vi "EditOptions.vi"(8 "error in":errorcluster, 11 "Fgen Instrument":refnum<class "Fgen Instrument.lvclass">) -> (0 "error out":errorcluster, 1 "edit options":T1, 2 "subnodes class":T2, 3 "Fgen Instrument out":refnum<class "Fgen Instrument.lvclass">)   [LabVIEW 2025, in "Fgen.lvlib" / "Fgen Instrument.lvclass"]
doc: "This VI Contains the options for the Menu that will be displayed when doing right click on an item\nThe subnodes class configures which nodes can be added to this nodes\nAnd the edit options determine which options are available for the node.\n\nThis configuration is stored in this VI in case some dynamic configuration is required for the menu options or subnodes.\n\nAll VIs must overide this methodCopyright 2017 National Instruments Corporation\n\nLicensed under the Apache License, Version 2.0 (the \"License\"); you may not use this file except in compliance with the License. You may obtain a copy of the License at http://www.apache.org/licenses/LICENSE-2.0\nUnless required by applicable law or agreed to in writing, software distributed under the License is distributed on an \"AS IS\" BASIS, WITHOUT WARRANTIES OR CONDITIONS OF ANY KIND, either express or implied. See the License for the specific language governing permissions and limitations under the License."
uses:
  Fgen Instrument.lvclass
  Users/Public/Documents/Sandia National Labs/TSS Plugin/CEF.lvlibp/Node/SubNodeCluster.ctl
  Users/Public/Documents/Sandia National Labs/TSS Plugin/CEF.lvlibp/Node/NodeMenuOptions.ctl
  Users/Public/Documents/Sandia National Labs/TSS Plugin/CEF.lvlibp/Node/CEF_Node.lvclass
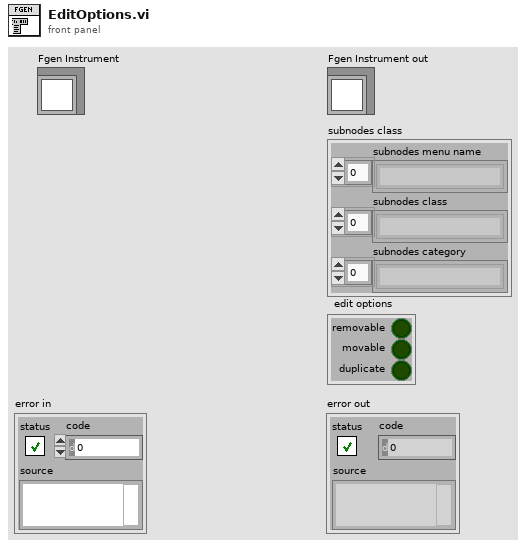
[diagram p1: front panel]
types:
  T1 = typedef "CEF.lvlibp/CEF_Node.lvclass/NodeMenuOptions.ctl" = cluster{"removable":bool, "movable":bool, "duplicate":bool}
  T2 = typedef "CEF.lvlibp/CEF_Node.lvclass/SubNodeCluster.ctl" = cluster{"subnodes menu name":string[], "subnodes class":string[], "subnodes category":string[]}
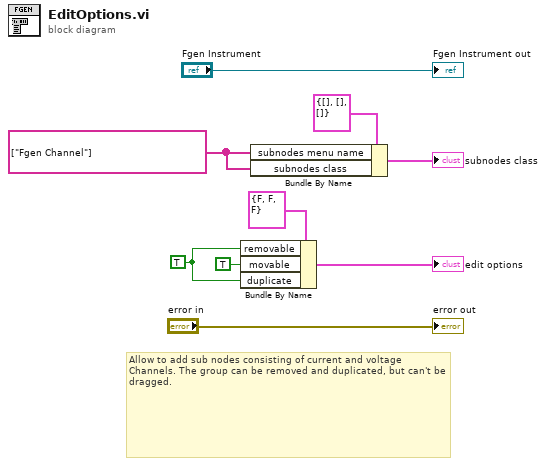
[diagram p0: block diagram]
diagram:
  w7 = TRUE ("movable")
  w2 = string[] ["Fgen Channel"] ("subnodes class")
  # "Allow to add sub nodes consisting of current and voltage Channels. The group can be removed and duplicated, but can't be dragged."
  n1 = Bundle By Name(cluster=T1 {"removable"=FALSE, "movable"=FALSE, "duplicate"=FALSE} ("edit options 2"), "removable"=w7, "movable"=TRUE, "duplicate"=w7) -> (→"edit options":T1)
  n2 = Bundle By Name(cluster=T2 {"subnodes menu name"=[], "subnodes class"=[], "subnodes category"=[]} ("subnodes class"), "subnodes menu name"=w2, "subnodes class"=w2) -> (→"subnodes class":T2)
  "error out" <- "error in"
  "Fgen Instrument out" <- "Fgen Instrument"
